vi "CMD_Drive.vi"(1 "Line":string) -> (0 "Done":bool)   [LabVIEW 2017, in "Apple script.lvlib"]
uses:
  Apple script.lvlib
  Robot Global Data.vi
  <vilib>/Rock Robotics/Network Tables/NT Write Numeric Array.vi
  <vilib>/addons/control/pid/pid.llb/PID (DBL).vi
  <vilib>/addons/control/pid/NI_PID_pid.lvlib
panel:
  in  "Subcommands":string[](array[string])=["at", "for", "until", "to", "stop", "reset"]
  in  "Parameters":i32[](array[numeric])=[2, 1, 1, 2, 0, 0]
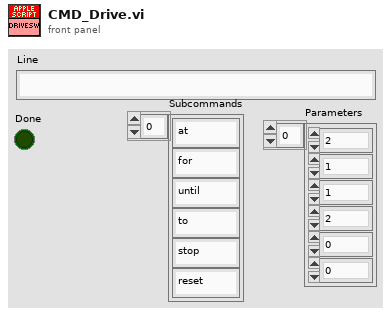
[diagram p1: front panel]
types:
  T1 = cluster{"proportional gain (Kc)":dbl, "integral time (Ti, min)":dbl, "derivative time (Td, min)":dbl}
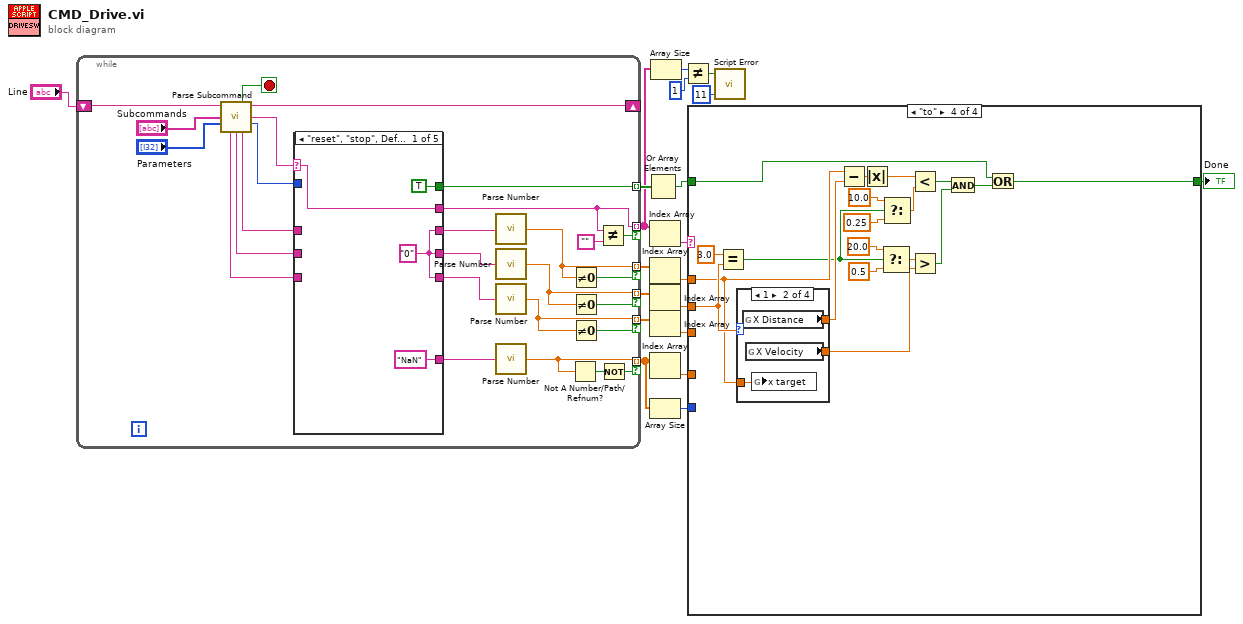
[diagram p0: block diagram]
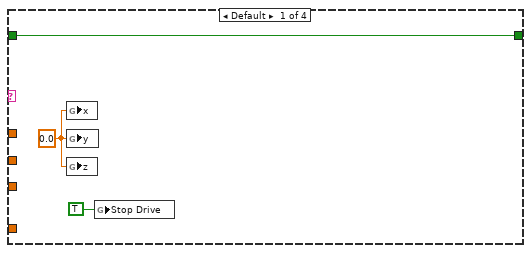
[diagram p2: hidden frame]
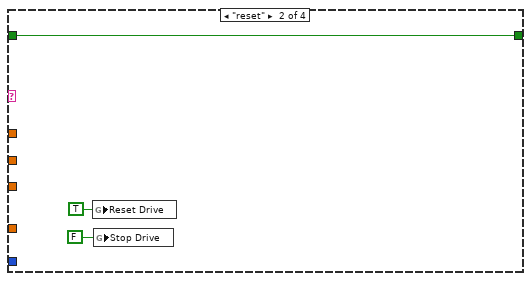
[diagram p3: hidden frame]
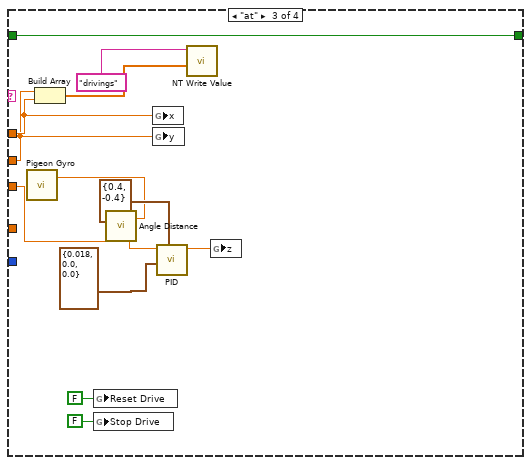
[diagram p4: hidden frame]
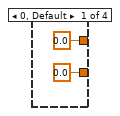
[diagram p5: hidden frame]
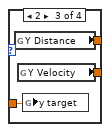
[diagram p6: hidden frame]
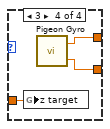
[diagram p7: hidden frame]
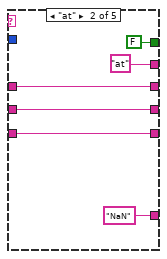
[diagram p8: hidden frame]
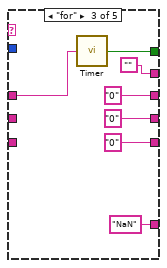
[diagram p9: hidden frame]
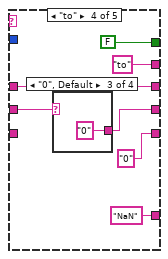
[diagram p10: hidden frame]
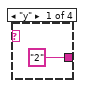
[diagram p11: hidden frame]
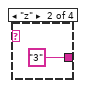
[diagram p12: hidden frame]
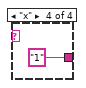
[diagram p13: hidden frame]
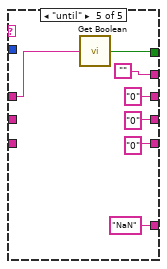
[diagram p14: hidden frame]
diagram:
  n1 = while {
    shift-right: [w43] -> _
    shift-left: "Line" -> [w46]
    tunnel: [w22] -> w9 mode=indexing
    tunnel: [w33] -> w17 mode=indexing if=w28
    tunnel: [w20] -> w16 mode=indexing if=w26
    tunnel: [w30] -> w15 mode=indexing if=w27
    tunnel: [w25] -> w7 mode=indexing if=w23
    tunnel: [w21] -> w8 mode=indexing if=w35
    stop <- w42 stop-if-true
    n2 = call "Parse Subcommand.vi"("Text In"=w46, "Subcommands"="Subcommands", "Parameters"="Parameters") -> ("Done"=w42:bool, "Text Out"=w43:string, "Subcommand"=w41:string, "# of Parameters"=w40:i32, "Parameter 3"=w38:string, "Parameter 2"=w37:string, "Parameter 1"=w39:string)  [unwired: 6 in]
    n3 = case shown="\"reset\", \"stop\", Default" w41 {
      selector: w41 -> [w47 _ _ _ _]
      tunnel: w40 -> [_ _ _ _ _]
      tunnel: w39 -> [_ w56 w57 w64 w76]
      tunnel: w37 -> [_ w55 _ w68 _]
      tunnel: w38 -> [_ w54 _ _ _]
      tunnel: [w49 w56 "0" ("Parameter 1") w68 "0" ("Parameter 1")] -> w34
      tunnel: [w49 w55 "0" ("Parameter 2") w67 "0" ("Parameter 1")] -> w32
      tunnel: [w49 w54 "0" ("Parameter 3") "0" ("Parameter 3") "0" ("Parameter 1")] -> w31
      tunnel: [TRUE ("Value") FALSE ("Running") w58 FALSE w75] -> w22
      tunnel: [w47 "at" "" "to" ("format string") ""] -> w21
      tunnel: ["NaN" ("Parameter 1") "NaN" ("Parameter 3") "NaN" ("Parameter 3") "NaN" ("Parameter 3") "NaN" ("Parameter 1")] -> w29
      frame "reset", "stop", Default {
        w49 = "0" ("format string")
      }
      frame "at" {
      }
      frame "for" {
        n4 = call "Timer.vi"("Seconds (string)"=w57) -> ("Done"=w58:bool)
      }
      frame "to" {
        n5 = case shown="\"0\", Default" w64 {
          tunnel: ["2" "3" "0" "1"] -> w67
          frame "y" {
          }
          frame "z" {
          }
          frame "0", Default {
          }
          frame "x" {
          }
        }
      }
      frame "until" {
        n6 = call "Get Boolean.vi"("Name"=w76) -> ("Value"=w75:bool)
      }
    }
    n7 = call "Parse Number.vi"("String"=w34) -> ("Number"=w33:dbl)
    n8 = call "Parse Number.vi"("String"=w32) -> ("Number"=w20:dbl)
    n9 = call "Parse Number.vi"("String"=w31) -> ("Number"=w30:dbl)
    n10 = call "Parse Number.vi"("String"=w29) -> ("Number"=w25:dbl)
    n11 = Not A Number/Path/Refnum?(number/path/refnum=w25) -> (NaN/Path/Refnum?=w24:bool)
    n12 = Not Equal To 0?(x=w33) -> (x != 0?=w28:bool)
    n13 = Not Equal To 0?(x=w20) -> (x != 0?=w26:bool)
    n14 = Not Equal To 0?(x=w30) -> (x != 0?=w27:bool)
    n15 = Not Equal?(x=w21, y="") -> (x != y?=w35:bool)
    n16 = Not(x=w24) -> (.not. x?=w23:bool)
  }
  n17 = Or Array Elements(Boolean array=w9) -> (logical OR=w2:bool)
  n18 = Index Array(array=w8) -> (element=w3:string)  [unwired: 1 in]
  n19 = Index Array(array=w17) -> (element=w1:dbl)  [unwired: 1 in]
  n20 = Index Array(array=w16) -> (element=w5:dbl)  [unwired: 1 in]
  n21 = Index Array(array=w15) -> (element=w14:dbl)  [unwired: 1 in]
  n22 = Index Array(array=w7) -> (element=w13:dbl)  [unwired: 1 in]
  n23 = Array Size(array=w7) -> (size(s)=w6:i32)
  n24 = Array Size(array=w8) -> (size(s)=w4:i32)
  n25 = Not Equal?(x=w4, y=1) -> (x != y?=w10:bool)
  n26 = case shown="\"to\"" w3 {
    tunnel: w1 -> [_ _ w93 w117]
    tunnel: w2 -> [w84 w87 w100 w101]
    tunnel: [w84 w87 w100 w102] -> w18
    tunnel: w5 -> [_ _ w92 w118]
    tunnel: w14 -> [_ _ w96 _]
    tunnel: w13 -> [_ _ _ _]
    tunnel: w6 -> [_ _ _ _]
    frame Default {
      w83 = 0.0 ("X")
      n27 = global write "Robot Global Data.vi" "x"(w83) -> ()
      n28 = global write "Robot Global Data.vi" "y"(w83) -> ()
      n29 = global write "Robot Global Data.vi" "z"(w83) -> ()
      n30 = global write "Robot Global Data.vi" "Stop Drive"(TRUE ("top rive")) -> ()
    }
    frame "reset" {
      n31 = global write "Robot Global Data.vi" "Reset Drive"(TRUE ("top rive")) -> ()
      n32 = global write "Robot Global Data.vi" "Stop Drive"(FALSE ("top rive")) -> ()
    }
    frame "at" {
      n33 = call "Pigeon Gyro.vi"() -> ("YPR.Yaw"=w97:dbl)  [unwired: 2 in, 1 out]
      n34 = Build Array(w92, w93) -> (w90:dbl[])
      n35 = global write "Robot Global Data.vi" "Reset Drive"(FALSE ("top rive")) -> ()
      n36 = global write "Robot Global Data.vi" "Stop Drive"(FALSE ("top rive")) -> ()
      n37 = call "Angle Distance.vi"("target angle"=w96, "current angle"=w97) -> ("distance"=w95:dbl)
      n38 = global write "Robot Global Data.vi" "x"(w93) -> ()
      n39 = global write "Robot Global Data.vi" "y"(w92) -> ()
      n40 = call-poly <vilib>:"PID.vi"("output range"=cluster{"output high":dbl, "output low":dbl} {"output high"=0.4, "output low"=-0.4}, "PID gains"=T1 {"proportional gain (Kc)"=0.018, "integral time (Ti, min)"=0.0, "derivative time (Td, min)"=0.0}, "setpoint"=w95) -> ("output"=w91:dbl)  [unwired: 7 in, 1 out]
      n41 = call-poly <vilib>:"NT Write Value.vi"("Numeric Array"=w90, "Name"="drivings") -> ()  [unwired: 9 in, 1 out]
      n42 = global write "Robot Global Data.vi" "z"(w91) -> ()
    }
    frame "to" {
      n43 = Equal?(x=3.0, y=w118) -> (x = y?=w106:bool)
      n44 = case shown="1" w118 {
        tunnel: [0.0 ("YPR.Yaw") w124 w127 w130] -> w112
        tunnel: [0.0 ("YPR.Yaw Rate") w123 w126 w129] -> w103
        tunnel: w117 -> [_ w122 w125 w128]
        frame 0, Default {
        }
        frame 1 {
          n45 = global read "Robot Global Data.vi" "X Distance"() -> (w124:dbl)
          n46 = global read "Robot Global Data.vi" "X Velocity"() -> (w123:dbl)
          n47 = global write "Robot Global Data.vi" "x target"(w122) -> ()
        }
        frame 2 {
          n48 = global read "Robot Global Data.vi" "Y Distance"() -> (w127:dbl)
          n49 = global read "Robot Global Data.vi" "Y Velocity"() -> (w126:dbl)
          n50 = global write "Robot Global Data.vi" "y target"(w125) -> ()
        }
        frame 3 {
          n51 = global write "Robot Global Data.vi" "z target"(w128) -> ()
          n52 = call "Pigeon Gyro.vi"() -> ("YPR.Yaw Rate"=w129:dbl, "YPR.Yaw"=w130:dbl)  [unwired: 2 in]
        }
      }
      n53 = Subtract(x=w117, y=w112) -> (x-y=w116:dbl)
      n54 = Absolute Value(x=w116) -> (abs(x)=w115:dbl)
      n55 = Select(t=20.0 ("y"), s=w106, f=0.5 ("y")) -> (s? t:f=w104:dbl)
      n56 = Select(t=10.0 ("y"), s=w106, f=0.25 ("y")) -> (s? t:f=w111:dbl)
      n57 = Less?(x=w115, y=w111) -> (x < y?=w113:bool)
      n58 = Greater?(x=w104, y=w103) -> (0:w114:bool)
      n59 = And(x=w113, y=w114) -> (x .and. y?=w119:bool)
      n60 = Or(x=w101, y=w119) -> (x .or. y?=w102:bool)
    }
  }
  "Done" <- w18
  n61 = call "Script Error.vi"("Error?"=w10, "Error Code"=11) -> ()  [unwired: 3 in, 1 out]
